vi "L_Delete_ZeroPoint.vi"(11 "Data in":T1(array[cluster])) -> (3 "Data out":T1(array[cluster]))   [LabVIEW 2019]
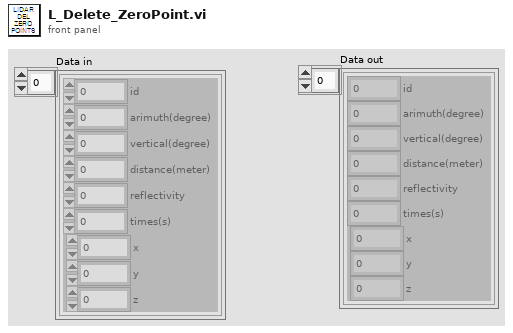
[diagram p1: front panel]
types:
  T1 = cluster{"id":i32, "arimuth(degree)":dbl, "vertical(degree)":dbl, "distance(meter)":dbl, "reflectivity":u8, "times(s)":ext, "x":dbl, "y":dbl, "z":dbl}[]
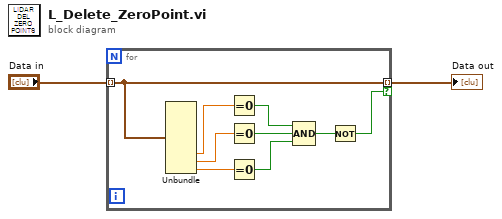
[diagram p0: block diagram]
diagram:
  n1 = for {
    tunnel: "Data in" -> [w11] mode=indexing
    tunnel: [w11] -> w1 mode=indexing if=w6
    n2 = Unbundle(w11) -> ("x"=w5:dbl, "y"=w4:dbl, "z"=w3:dbl)  [unwired: 6 out]
    n3 = Equal To 0?(x=w5) -> (x = 0?=w10:bool)
    n4 = Equal To 0?(x=w4) -> (x = 0?=w9:bool)
    n5 = Equal To 0?(x=w3) -> (x = 0?=w8:bool)
    n6 = Compound Arithmetic op=AND(w10, w9, w8) -> (w7:bool)
    n7 = Not(x=w7) -> (.not. x?=w6:bool)
  }
  "Data out" <- w1
